vi "SMTP Email EUC.vi"(11 "text":string) -> (2 "isEUC?":bool)   [LabVIEW 2012, in "NewNI_SMTPEmail.lvlib"]
uses:
  NewNI_SMTPEmail.lvlib
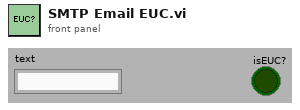
[diagram p1: front panel]
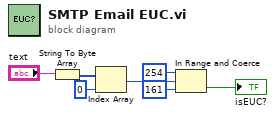
[diagram p0: block diagram]
diagram:
  n1 = String To Byte Array(string="text") -> (unsigned byte array=w6:u8[])
  n2 = Index Array(array=w6, index=0) -> (element=w4:u8)
  n3 = In Range and Coerce(upper limit=u8 254, x=w4, lower limit=u8 161) -> (In Range?=→"isEUC?":bool)  [unwired: 1 out]
